vi "GVZwangsMPV_ECD.vi"() -> ()   [LabVIEW 2017]
panel:
  out "ZwangsMPV?":bool
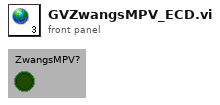
[diagram p1: front panel]
diagram:
